vi "Read current filename.vi"(8 "error in (no error)":errorcluster, 11 "Manage File Response in":refnum<class "Manage File Response.lvclass">) -> (0 "error out":errorcluster, 2 "current filename":path, 3 "Manage File Response out":refnum<class "Manage File Response.lvclass">)   [LabVIEW 2020, in "AIM ARINC 664 Engine.lvlib" / "Implementation.lvlib" / "Frame Logging.lvlib" / "Manage File Response.lvclass"]
uses:
  Manage File Response.lvclass
  Manage File Response.lvclass/Manage File Response.ctl
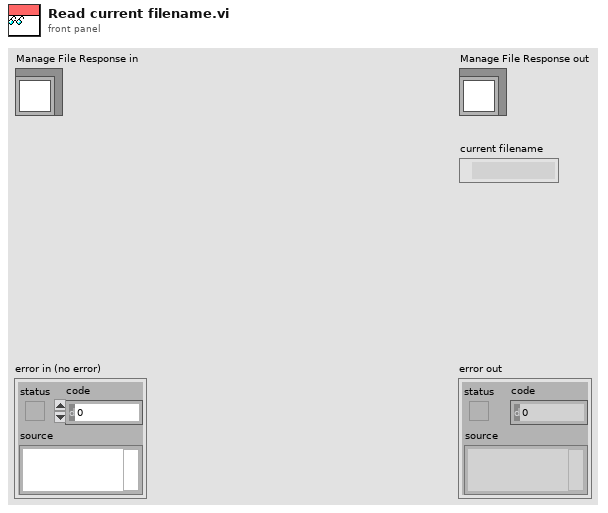
[diagram p1: front panel]
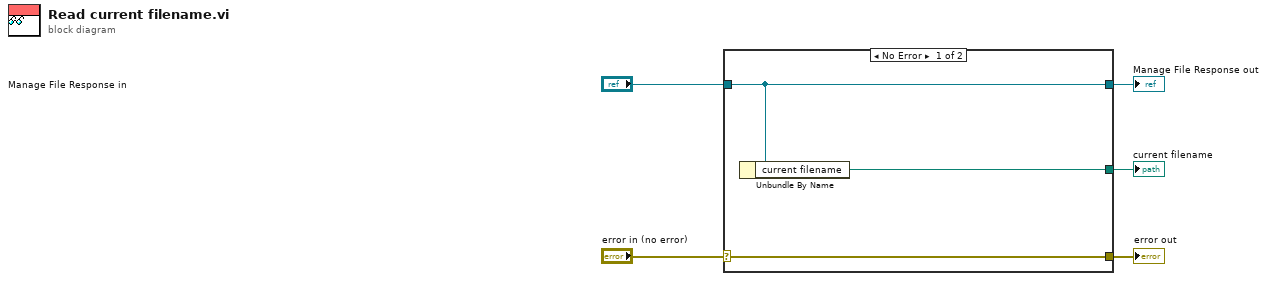
[diagram p0: block diagram]
diagram:
  n1 = case shown="No Error" "error in (no error)" {
    selector: "error in (no error)" -> [w8 w9]
    tunnel: [w8 w9] -> w4
    tunnel: [w7 w10] -> w2
    tunnel: "Manage File Response in" -> [w7 w10]
    tunnel: [w6 _] -> w1
    frame No Error {
      n2 = Unbundle By Name(w7) -> ("current filename"=w6:path)
    }
    frame Error {
    }
  }
  "error out" <- w4
  "Manage File Response out" <- w2
  "current filename" <- w1
